vi "LEBITplc.CreateServicesAndEvent.vi"(0 "i ref in":refnum<vi>, 5 "error in(no error)":errorcluster) -> (14 "i ref out":refnum<vi>, 19 "error out":errorcluster)   [LabVIEW 2014, in "LEBITplc.lvlib"]
doc: "This is the constructor of a class.\n\nLicense Agreement for this software:\n\nCopyright (C)\nGesellschaft für Schwerionenforschung, GSI\nPlanckstr. 1\n64291 Darmstadt\nGermany\n\nContact: D.Beck@gsi.de \n\nThis program is free software; you can redistribute it and/or modify it under the terms of the \nGNU General Public License as published by the Free Software Foundation; either version 2 of \nthe license, or (at your option) any later version.\n\nThis program is distributed in the hope that it will be useful, but WITHOUT ANY WARRANTY; \nwithout even the implied warranty of MERCHANTABILITY or FITNESS FOR A PARTICULAR PURPOSE. See the GNU General License for more details (http://www.gnu.org).\n\nGesellschaft für Schwerionenforschung, GSI\nPlanckstr. 1, 64291 Darmstadt, Germany\nFor all questions and ideas contact: M.Richter@gsi.de, H.Brand@gsi.de or D.Beck@gsi.de.\nLast update: 16-JUN-2004"
uses:
  LEBITplc.lvlib
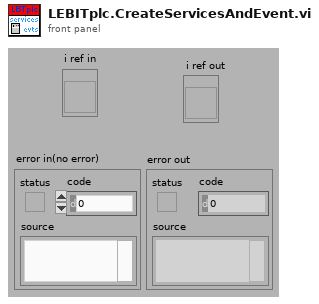
[diagram p1: front panel]
types:
  T1 = typedef "LEBITplc.lvlib/LEBITplc.i attribute.ctl" = cluster{"LLFLocation":string, "SetFileLocation":string, "nickNames":string[], "setValuePLCServiceID":i32[], "GUIServiceID":i32[], "monValuePLC":string[], "SetValueServiceID":i32[], "MonValueServiceID":i32[], "SetValue":dbl[][], "SetValueMin":dbl[], "SetValueMax":dbl[], "SetValueInfoServiceID":i32[], "GUINames":string[], "ListOfBases":string[], "Scale":dbl[], "Offset":dbl[], "setValuePLC":string[], "BaseName":string[], "ScaleServiceID":i32[], "OffsetServiceID":i32[], "AllPLCValues":string[], "CondSpecialArray":string[][], "CondSpecialIndex":i32[], "CondSpecialMonValue":dbl[], "RecentlyChanged":i32[], "SetFileLocationID":i32, "Dependent-Monitors":string[][], "LastLoadedFiles":string[], "IonGuideCalibLocation":string, "Monitor Dependent":string[], "Special":string[], "PLC?":bool[], "Start Date":string, "ListOfBasesServiceID":i32, "SETRA VISA resource":refnum<visa-resource-name>}
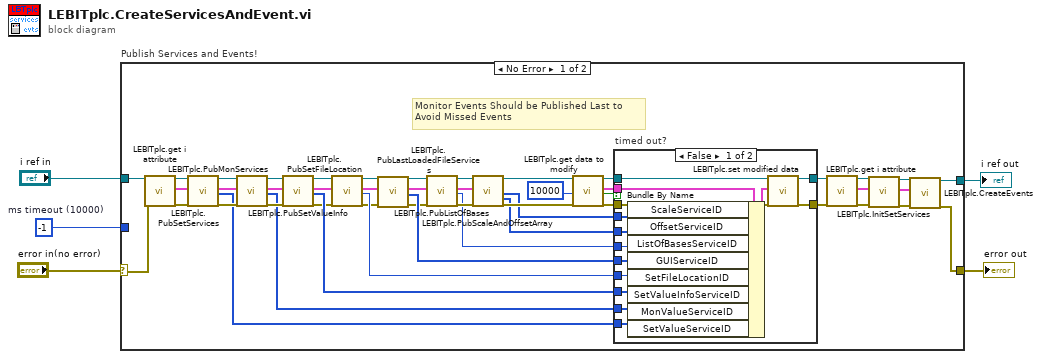
[diagram p0: block diagram]
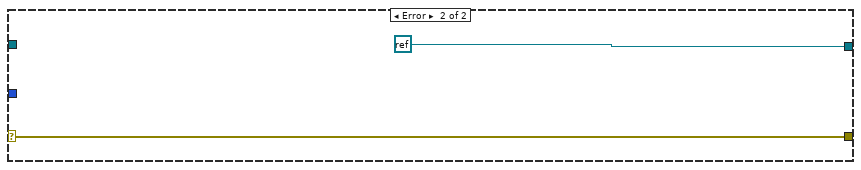
[diagram p3: hidden frame]
diagram:
  w1 = -1  # ms timeout (10000)
  n1 = case "Publish Services and Events!" shown="No Error" "error in(no error)" {
    selector: "error in(no error)" -> [w52 w71]
    tunnel: [w19 w71] -> w5
    tunnel: "i ref in" -> [w53 _]
    tunnel: [w20 refnum<k0> refnum] -> w2
    tunnel: w1 -> [_ _]
    frame No Error {
      # "Monitor Events Should be Published Last to\nAvoid Missed Events"
      n2 = call "LEBITplc.get i attribute.vi"("i ref in"=w53, "error in (no error)"=w52) -> ("i ref out"=w51:refnum<vi>, "i attribute"=w43:T1, "error out"=w50:errorcluster)  [unwired: 15 in]
      n3 = call "LEBITplc.PubSetServices.vi"("i ref in"=w51, "i attribute in"=w43, "error in"=w50) -> ("i ref out"=w49:refnum<vi>, "i attribute out"=w42:T1, "SetValueServiceID"=w37:i32[], "error out"=w48:errorcluster)  [unwired: 13 in]
      n4 = call "LEBITplc.PubMonServices.vi"("i ref in"=w49, "i attribute in"=w42, "error in"=w48) -> ("i ref out"=w40:refnum<vi>, "i attribute out"=w38:T1, "MonValueServiceID"=w36:i32[], "error out"=w39:errorcluster)  [unwired: 13 in]
      n5 = call "LEBITplc.PubSetValueInfo.vi"("i ref in"=w40, "i attribute in"=w38, "error in"=w39) -> ("i ref out"=w18:refnum<vi>, "i attribute out"=w17:T1, "SetValueInfoServiceID"=w28:i32[], "error out"=w16:errorcluster)  [unwired: 13 in]
      n6 = call "LEBITplc.PubSetFileLocation.vi"("i ref in"=w18, "i attribute in"=w17, "error in"=w16) -> ("i ref out"=w13:refnum<vi>, "i attribute out"=w12:T1, "SetFileLocationID"=w15:i32, "error out"=w11:errorcluster)  [unwired: 13 in]
      n7 = call "LEBITplc.PubLastLoadedFileServices.vi"("i ref in"=w13, "i attribute in"=w12, "error in"=w11) -> ("i ref out"=w7:refnum<vi>, "i attribute out"=w8:T1, "GUIServiceID"=w10:i32[], "error out"=w9:errorcluster)  [unwired: 13 in]
      n8 = call "LEBITplc.PubListOfBases.vi"("i ref in"=w7, "i attribute in"=w8, "error in"=w9) -> ("i ref out"=w34:refnum<vi>, "i attribute out"=w35:T1, "List of Bases serviceID"=w6:i32, "error out"=w33:errorcluster)  [unwired: 13 in]
      n9 = call "LEBITplc.PubScaleAndOffsetArray.vi"("i ref in"=w34, "i attribute in"=w35, "error in"=w33) -> ("i ref out"=w32:refnum<vi>, "ScaleServiceID"=w30:i32[], "OffsetServiceID"=w29:i32[], "error out"=w31:errorcluster)  [unwired: 12 in, 1 out]
      n10 = call "LEBITplc.get data to modify.vi"("i ref in"=w32, "ms timeout (10000)"=10000, "error in (no error)"=w31) -> ("i ref out"=w46:refnum<vi>, "i attribute"=w44:T1, "timed out"=w47:bool, "error out"=w45:errorcluster)  [unwired: 13 in]
      n11 = case "timed out?" shown="False" w47 {
        tunnel: [w67 w69] -> w27
        tunnel: [w66 w68] -> w26
        tunnel: w46 -> [w65 w69]
        tunnel: w45 -> [w64 w68]
        tunnel: w44 -> [w63 _]
        tunnel: w37 -> [w61 _]
        tunnel: w36 -> [w60 _]
        tunnel: w28 -> [w57 _]
        tunnel: w30 -> [w59 _]
        tunnel: w29 -> [w58 _]
        tunnel: w10 -> [w55 _]
        tunnel: w15 -> [w56 _]
        tunnel: w6 -> [w54 _]
        frame False {
          n12 = Bundle By Name(cluster=w63, "ScaleServiceID"=w59, "OffsetServiceID"=w58, "ListOfBasesServiceID"=w54, "GUIServiceID"=w55, "SetFileLocationID"=w56, "SetValueInfoServiceID"=w57, "MonValueServiceID"=w60, "SetValueServiceID"=w61) -> (w62:T1)
          n13 = call "LEBITplc.set modified data.vi"("i ref in"=w65, "i attribute"=w62, "error in (no error)"=w64) -> ("i ref out"=w67:refnum<vi>, "error out"=w66:errorcluster)  [unwired: 15 in]
        }
        frame True {
        }
      }
      n14 = call "LEBITplc.get i attribute.vi"("i ref in"=w27, "error in (no error)"=w26) -> ("i ref out"=w25:refnum<vi>, "i attribute"=w24:T1, "error out"=w14:errorcluster)  [unwired: 15 in]
      n15 = call "LEBITplc.InitSetServices.vi"("i ref in"=w25, "i attribute in"=w24, "error in"=w14) -> ("i ref out"=w23:refnum<vi>, "i attribute out"=w22:T1, "error out"=w21:errorcluster)  [unwired: 14 in]
      n16 = call "LEBITplc.CreateEvents.vi"("i ref in"=w23, "i attribute in"=w22, "error in"=w21) -> ("i ref out"=w20:refnum<vi>, "error out"=w19:errorcluster)  [unwired: 14 in, 1 out]
    }
    frame Error {
    }
  }
  "i ref out" <- w2
  "error out" <- w5
